vi "test Blob and Container Metadata.vi"(8 "error in (no error)":errorcluster, 11 "TestCase in":refnum<class "Test_Blob.lvclass">) -> (0 "error out":errorcluster, 3 "TestCase out":refnum<class "Test_Blob.lvclass">)   [LabVIEW 2015, in "Test_Blob.lvclass"]
uses:
  Test_Blob.lvclass
  Blob Storage/Blob Type.ctl
  Core/Name Value Pair.ctl
  Global Parameters.vi
  Core/Session/Session.lvclass
  Blob Storage/NI_Azure_Blob.lvlib
  Core/NI_Azure_Core.lvlib
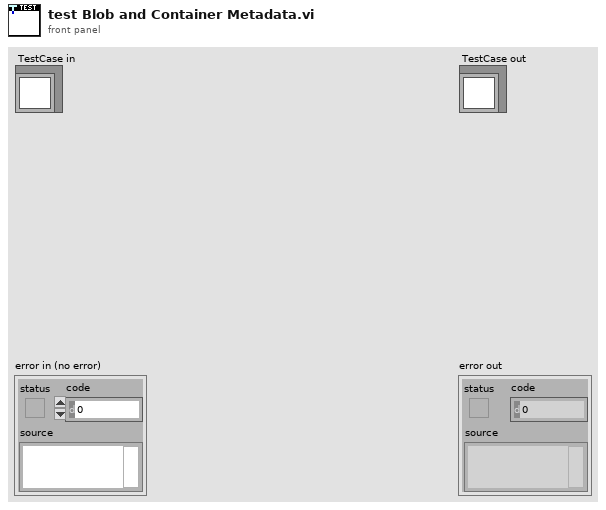
[diagram p1: front panel]
types:
  T1 = typedef "NI_Azure_Core.lvlib/Name Value Pair.ctl" = cluster{"name":string, "value":string}
  T2 = typedef "NI_Azure_Blob.lvlib/Blob Type.ctl" = enum16{"BlockBlob", "PageBlob", "AppendBlob"}
  T3 = typedef "NI_Azure_Core.lvlib/Azure Credentials.ctl" = cluster{"Storage Account Name":string, "Access Key":string}
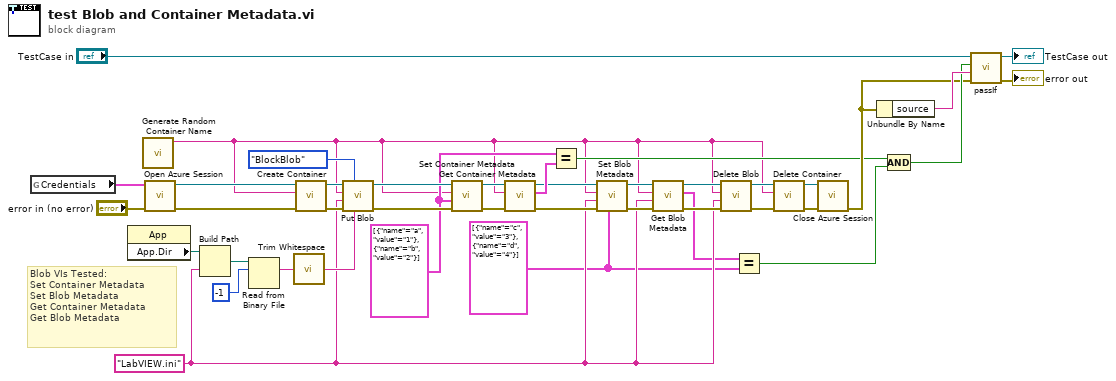
[diagram p0: block diagram]
diagram:
  w3 = T1[] [{"name"="c", "value"="3"}, {"name"="d", "value"="4"}] ("Metadata")
  w12 = T1[] [{"name"="a", "value"="1"}, {"name"="b", "value"="2"}] ("Metadata")
  w4 = "LabVIEW.ini"
  # "Blob VIs Tested:\nSet Container Metadata\nSet Blob Metadata\nGet Container Metadata\nGet Blob Metadata"
  n1 = global read "Global Parameters.vi" "Credentials"() -> (w25:T3)
  n2 = property class="App"() -> ("App.Dir"=w36:path)  [unwired: 2 in, 2 out]
  n3 = call "Generate Random Container Name.vi"() -> ("Random Container Name"=w5:string)  [unwired: 11 in]
  n4 = call "Open Azure Session.vi"("error in (no error)"="error in (no error)", "Credentials"=w25) -> ("error out"=w26:errorcluster, "Azure Session"=w22:refnum<class "Session.lvclass">)  [unwired: 8 in]
  n5 = Build Path(base path=w36, name or relative path=w4) -> (appended path=w35:path)
  n6 = Read from Binary File(10:-1 ("count (1)"), 11:w35) -> (2:w30:string)  [unwired: 4 in, 3 out]
  n7 = call <vilib>:"Trim Whitespace.vi"("string"=w30) -> ("trimmed string"=w21:string)  [unwired: 1 in]
  n8 = call "Create Container.vi"("error in (no error)"=w26, "Container"=w5, "Azure Session in"=w22) -> ("error out"=w33:errorcluster, "Azure Session out"=w32:refnum<class "Session.lvclass">)  [unwired: 7 in]
  n9 = call "Put Blob.vi"("Blob Content"=w21, "Blob type"=Blob_Type."BlockBlob", "error in (no error)"=w33, "Blob"=w4, "Container"=w5, "Azure Session in"=w32) -> ("error out"=w31:errorcluster, "Azure Session out"=w16:refnum<class "Session.lvclass">)  [unwired: 4 in]
  n10 = call "Set Container Metadata.vi"("error in (no error)"=w31, "Metadata"=w12, "Container"=w5, "Azure Session in"=w16) -> ("error out"=w17:errorcluster, "Azure Session out"=w14:refnum<class "Session.lvclass">)  [unwired: 6 in]
  n11 = call "Get Container Metadata.vi"("error in (no error)"=w17, "Container"=w5, "Azure Session in"=w14) -> ("error out"=w15:errorcluster, "Metadata"=w13:T1[], "Azure Session out"=w9:refnum<class "Session.lvclass">)  [unwired: 6 in]
  n12 = Equal?(x=w12, y=w13) -> (x = y?=w11:bool)
  n13 = call "Set Blob Metadata.vi"("Blob Metadata"=w3, "error in (no error)"=w15, "Blob"=w4, "Container"=w5, "Azure Session in"=w9) -> ("error out"=w10:errorcluster, "Azure Session out"=w7:refnum<class "Session.lvclass">)  [unwired: 5 in]
  n14 = call "Get Blob Metadata.vi"("error in (no error)"=w10, "Blob"=w4, "Container"=w5, "Azure Session in"=w7) -> ("error out"=w8:errorcluster, "Blob Metadata"=w2:T1[], "Azure Session out"=w6:refnum<class "Session.lvclass">)  [unwired: 5 in]
  n15 = call "Delete Blob.vi"("error in (no error)"=w8, "Blob"=w4, "Container"=w5, "Azure Session in"=w6) -> ("error out"=w29:errorcluster, "Azure Session out"=w28:refnum<class "Session.lvclass">)  [unwired: 6 in]
  n16 = Equal?(x=w2, y=w3) -> (x = y?=w1:bool)
  n17 = call "Delete Container.vi"("error in (no error)"=w29, "Container"=w5, "Azure Session in"=w28) -> ("error out"=w24:errorcluster, "Azure Session out"=w18:refnum<class "Session.lvclass">)  [unwired: 7 in]
  n18 = call "Close Azure Session.vi"("error in (no error)"=w24, "Azure Session"=w18) -> ("error out"=w19:errorcluster)  [unwired: 9 in]
  n19 = Unbundle By Name(w19) -> ("source"=w37:string)
  n20 = Compound Arithmetic op=AND(w11, w1) -> (w23:bool)
  n21 = call-dynamic "passIf.vi"("error in (no error)"=w19, "message (\"\")"=w37, "pass"=w23, "TestCase in"="TestCase in") -> ("error out"=→"error out":errorcluster, "TestCase out"=→"TestCase out":refnum<class "Test_Blob.lvclass">)  [unwired: 6 in]
